vi "Pre Launch Init.vi"(11 "Main_UI in":refnum<class "Main_UI.lvclass">) -> (0 "error out":errorcluster, 3 "Main_UI out":refnum<class "Main_UI.lvclass">)   [LabVIEW 2020, in "Main_UI.lvlib" / "Main_UI.lvclass"]
doc: "(<B>Filename</B>: Actor Framework.lvlib:Actor.lvclass:Pre Launch Init.vi)\n\nDefines behavior that occurs after the Launch Nested Actor method is invoked but before the actor's Actor Core method begins running.\n\nBy default, this method does nothing. A descendant class may override it to define behavior."
uses:
  Main_UI.lvclass
  Main_UI.lvclass/Main_UI.ctl
  <vilib>/ActorFramework/Actor/Actor.lvclass
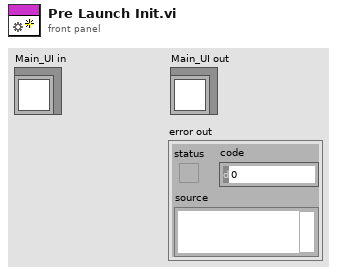
[diagram p1: front panel]
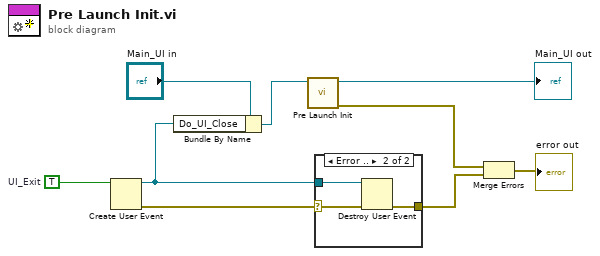
[diagram p0: block diagram]
diagram:
  w8 = TRUE  # UI_Exit
  n1 = Create User Event(user event datatype=w8) -> (user event=w4:refnum<user-event>, error out=w5:errorcluster)  [unwired: 1 in]
  n2 = Bundle By Name(cluster="Main_UI in", "Do_UI_Close"=w4) -> (w6:refnum<class "Main_UI.lvclass">)
  n3 = call-parent "Pre Launch Init.vi"("Actor in"=w6) -> ("error out"=w2:errorcluster, "Actor out"=→"Main_UI out":refnum<class "Main_UI.lvclass">)  [unwired: 9 in]
  n4 = case shown="Error .." w5 {
    selector: w5 -> [w10 w12]
    tunnel: [w10 w13] -> w1
    tunnel: w4 -> [_ w11]
    frame No Error {
    }
    frame Error {
      n5 = Destroy User Event(user event=w11, error in=w12) -> (error out=w13:errorcluster)
    }
  }
  n6 = Merge Errors(w2, w1) -> (→"error out":errorcluster)
